vi "Startup.vi"(7 "App":refnum<class>, 8 "error in (no error)":errorcluster, 10 "Config":refnum<class>, 11 "Temp01 in":refnum<class "TELLC_Temp01.lvclass">) -> (0 "error out":errorcluster, 3 "Temp01 out":refnum<class "TELLC_Temp01.lvclass">)   [LabVIEW 2017, in "TELLC_Temp01.lvclass"]
doc: "Developed by Kevin Thompson\nkevin@thompsonengineering.net\n\nCopyright 2018\nThompson Engineering, LLC"
uses:
  TELLC_Temp01.lvclass
  DataTypes/Dependency--cluster.ctl
  TELLC_Temp01.lvclass/TELLC_Temp01.ctl
  Accessors/Set Dependency.vi
  Accessors/Set VISA Ref.vi
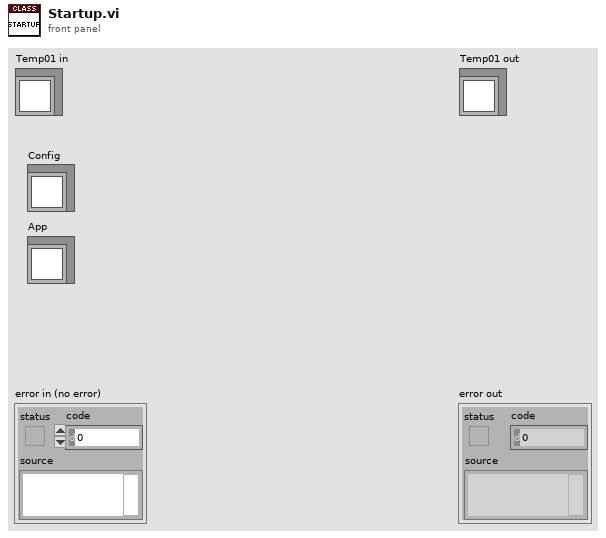
[diagram p1: front panel]
types:
  T1 = typedef "TELLC_Temp01.lvclass/Dependency--cluster.ctl" = cluster{"Config":refnum<class>, "ClassRef":refnum<class>}
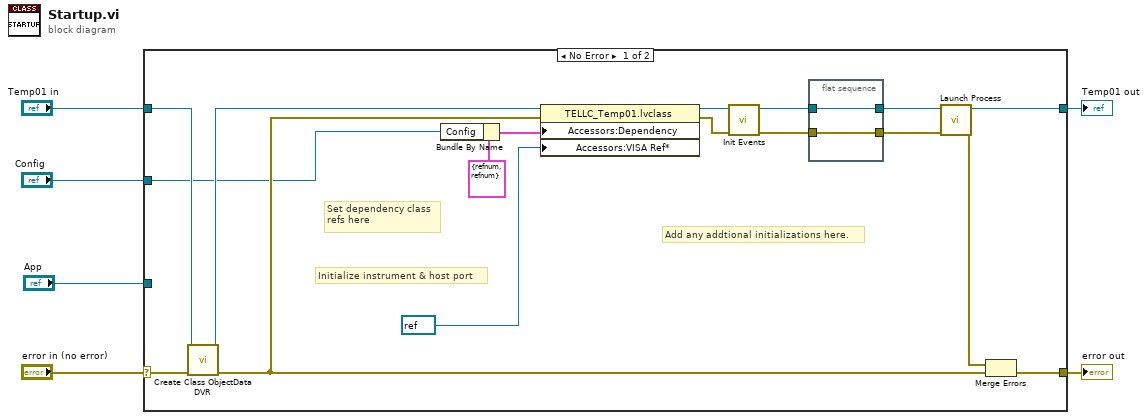
[diagram p0: block diagram]
diagram:
  n1 = case shown="No Error" "error in (no error)" {
    selector: "error in (no error)" -> [w23 w27]
    tunnel: [w16 w27] -> w5
    tunnel: [w13 w26] -> w3
    tunnel: "Temp01 in" -> [w21 w26]
    tunnel: "Config" -> [w8 _]
    tunnel: "App" -> [_ _]
    frame No Error {
      # "Set dependency class\nrefs here"
      # "Initialize instrument & host port"
      # "Add any addtional initializations here."
      n2 = call "Create Class ObjectData DVR.vi"("error in (no error)"=w23, "Temp01 in"=w21) -> ("error out"=w11:errorcluster, "Temp01 out"=w20:refnum<class "TELLC_Temp01.lvclass">)  [unwired: 8 in]
      n3 = Bundle By Name(cluster=T1 {"Config"=refnum, "ClassRef"=refnum} ("Dependency"), "Config"=w8) -> (w7:T1)
      n4 = property class="TELLC_Temp01.lvclass"(reference=w20, error in=w11, "Accessors:Dependency"=w7, "Accessors:VISA Ref*"=refnum<visa-resource-name> refnum ("VISA Ref*")) -> (reference out=w22:refnum<class "TELLC_Temp01.lvclass">, error out=w19:errorcluster)
      n5 = call "Init Events.vi"("error in (no error)"=w19, "Temp01 in"=w22) -> ("error out"=w17:errorcluster, "Temp01 out"=w18:refnum<class "TELLC_Temp01.lvclass">)  [unwired: 8 in]
      n6 = flat-sequence {
        tunnel: w18 -> [w25]
        tunnel: [w25] -> w14
        tunnel: w17 -> [w24]
        tunnel: [w24] -> w15
        frame #0 {
        }
      }
      n7 = call "Launch Process.vi"("error in (no error)"=w15, "Temp01 in"=w14) -> ("error out"=w12:errorcluster, "Temp01 out"=w13:refnum<class "TELLC_Temp01.lvclass">)  [unwired: 6 in, 2 out]
      n8 = Merge Errors(w12, w11) -> (w16:errorcluster)
    }
    frame Error {
    }
  }
  "error out" <- w5
  "Temp01 out" <- w3
